vi "poly_data_queue_ArrayEXT.vi"(5 "skip? (F)":bool, 6 "initial queue element (vector of NaNs)":ext[](array[numeric]), 7 "initialize":bool, 8 "error in":errorcluster caption="Error in (no error)", 9 "queue length (100)":i32=100, 10 "input data element":ext[](array[numeric]) format="%0.2f") -> (0 "error out":errorcluster, 1 "eliminated element":ext[](array[numeric]) format="%0.2f", 2 "queue":ext[][](array[numeric]), 4 "current length":i32)   [LabVIEW 2015]
uses:
  poly_average_tools_eco_plus.vi
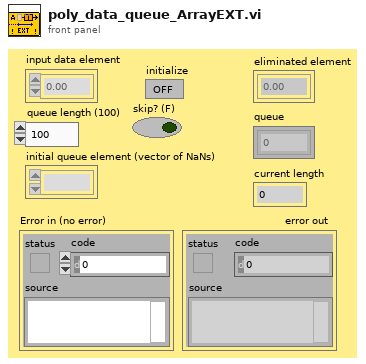
[diagram p1: front panel]
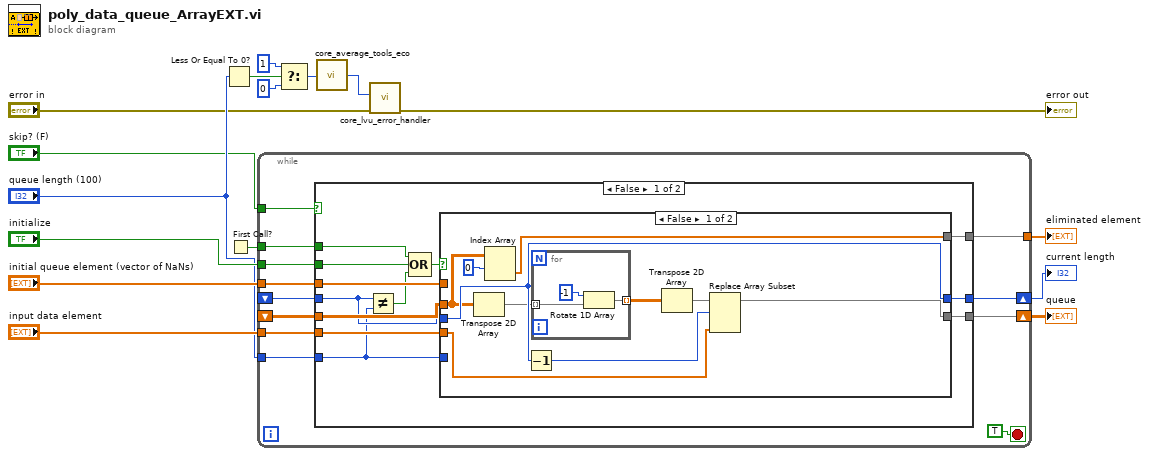
[diagram p0: block diagram]
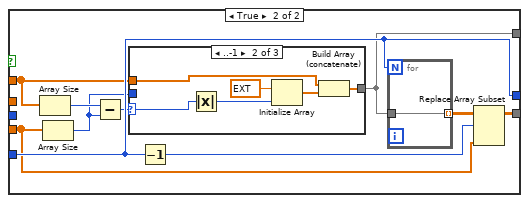
[diagram p2: hidden frame]
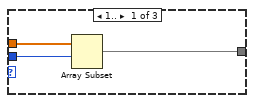
[diagram p3: hidden frame]
diagram:
  n1 = Less Or Equal To 0?(x="queue length (100)") -> (x <= 0?=w9:bool)
  n2 = First Call?() -> (First Call?: T/F=w10:bool)
  n3 = while {
    tunnel: w10 -> [w23]
    shift-left: _ -> [w26]
    shift-right: [w27] -> w16
    shift-left: _ -> [w25]
    shift-right: [w28] -> w4
    tunnel: "initialize" -> [w22]
    tunnel: "input data element" -> [w21]
    tunnel: "initial queue element (vector of NaNs)" -> [w20]
    tunnel: "queue length (100)" -> [w19]
    tunnel: [w18] -> w12
    tunnel: "skip? (F)" -> [w17]
    stop <- TRUE stop-if-true
    n4 = case shown="False" w17 {
      tunnel: [w40 w77] -> w28
      tunnel: [w39 w75] -> w27
      tunnel: w26 -> [w30 w75]
      tunnel: w25 -> [w38 w77]
      tunnel: w23 -> [w33 _]
      tunnel: w22 -> [w32 _]
      tunnel: w21 -> [w37 w76]
      tunnel: w20 -> [w36 _]
      tunnel: w19 -> [w29 _]
      tunnel: [w35 w76] -> w18
      frame False {
        n5 = Not Equal?(x=w30, y=w29) -> (x != y?=w34:bool)
        n6 = Compound Arithmetic op=OR(w33, w32, w34) -> (w31:bool)
        n7 = case shown="False" w31 {
          tunnel: [w48 w62] -> w40
          tunnel: [w49 w61] -> w39
          tunnel: w30 -> [w49 _]
          tunnel: w38 -> [w42 _]
          tunnel: w37 -> [w50 w59]
          tunnel: w36 -> [_ w58]
          tunnel: w29 -> [_ w61]
          tunnel: [w45 w57] -> w35
          frame False {
            n8 = Transpose 2D Array(2D array=w42) -> (transposed array=w44:ext[][])
            n9 = Index Array(array=w42, index (row)=0 ("Index")) -> (element=w45:ext[])  [unwired: 1 in]
            n10 = Decrement(x=w49) -> (x-1=w47:i32)
            n11 = for {
              tunnel: w44 -> [w53] mode=indexing
              tunnel: [w52] -> w43 mode=indexing
              n12 = Rotate 1D Array(1:w53, 2:i16 -1 ("n")) -> (0:w52:ext[])
            }
            n13 = Transpose 2D Array(2D array=w43) -> (transposed array=w41:ext[][])
            n14 = Replace Array Subset(array=w41, new element=w50, index (row)=w47) -> (w48:ext[][])  [unwired: 1 in]
          }
          frame True {
            n15 = Array Size(array=w58) -> (size(s)=w56:i32)
            n16 = Array Size(array=w59) -> (size(s)=w54:i32)
            n17 = Subtract(x=w56, y=w54) -> (x-y=w55:i32)
            n18 = case shown="..-1" w55 {
              selector: w55 -> [_ w72 _]
              tunnel: [w64 w67 w73] -> w57
              tunnel: w58 -> [w66 w69 w73]
              tunnel: w54 -> [w65 _ _]
              frame 1.. {
                n19 = Array Subset(array=w66, index=w65) -> (w64:ext[])  [unwired: 1 in]
              }
              frame ..-1 {
                n20 = Absolute Value(x=w72) -> (abs(x)=w71:i32)
                n21 = Initialize Array(ext nan ("element"), w71) -> (w68:ext[])
                n22 = Build Array (concatenate)(w69, w68) -> (w67:ext[])
              }
              frame 0 {
              }
            }
            n23 = Decrement(x=w61) -> (x-1=w63:i32)
            n24 = for {
              N: w61 -> [_]
              tunnel: w57 -> [w74]
              tunnel: [w74] -> w60 mode=indexing
            }
            n25 = Replace Array Subset(array=w60, new element=w59, index (row)=w63) -> (w62:ext[][])  [unwired: 1 in]
          }
        }
      }
      frame True {
      }
    }
  }
  "queue" <- w4
  "current length" <- w16
  "eliminated element" <- w12
  n26 = Select(t=1, s=w9, f=0) -> (s? t:f=w2:i32)
  n27 = call-poly "core_average_tools_eco.vi"("code (w/out eco)"=w2) -> ("code (+ eco)"=w1:i32)  [unwired: 4 in]
  n28 = call "core_lvu_error_handler.vi"("error in (no error)"="error in", "code (0 = no error)"=w1) -> ("error out"=→"error out":errorcluster)  [unwired: 8 in, 1 out]
